vi "RaiseErrorIf.vi"(8 "error in (no error)":errorcluster, 9 "error message":string, 10 "error code (5888)":i32=5888 format="%0.0f", 11 "error? (true)":bool=TRUE) -> (0 "error out":errorcluster)   [LabVIEW 2020]
uses:
  <vilib>/Utility/error.llb/DialogType.ctl
panel:
  # "error? が true のときにエラーを生じる\n（ダイアログは出さない）\n任意のメッセージを指定できる\n（発生元情報が追加される）\nコードはデフォルトで 5888 になる"
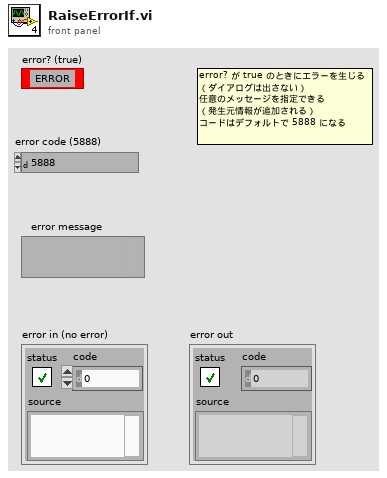
[diagram p1: front panel]
types:
  T1 = typedef "DialogType.ctl" = u16
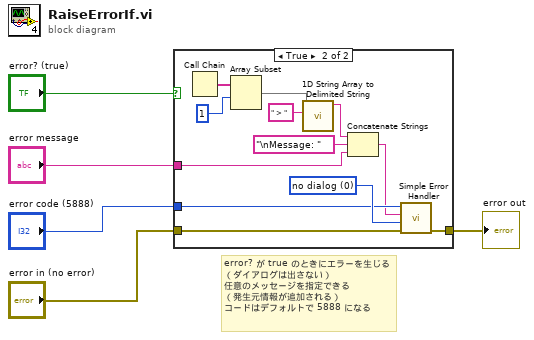
[diagram p0: block diagram]
diagram:
  # "error? が true のときにエラーを生じる\n（ダイアログは出さない）\n任意のメッセージを指定できる\n（発生元情報が追加される）\nコードはデフォルトで 5888 になる"
  n1 = case shown="True" "error? (true)" {
    tunnel: "error in (no error)" -> [w6 w18]
    tunnel: [w6 w17] -> w4
    tunnel: "error message" -> [_ w11]
    tunnel: "error code (5888)" -> [_ w15]
    frame False {
    }
    frame True {
      w16 = T1 0 items=["no dialog", "OK message", "continue or stop message", "OK message + warnings", "continue/stop + warnings"] ("type of dialog (OK msg:1)")
      n2 = Call Chain() -> (call chain=w9:string[])
      n3 = Array Subset(array=w9, index=1) -> (w7:string[])  [unwired: 1 in]
      n4 = call <vilib>:"1D String Array to Delimited String.vi"("delimiter"=" > ", "string array"=w7) -> ("delimited string"=w13:string)  [unwired: 9 in]
      n5 = Concatenate Strings(w13, "\nMessage: " ("string"), w11) -> (w10:string)
      n6 = call <vilib>:"Simple Error Handler.vi"("error code (no error:0)"=w15, "error source (\" \")"=w10, "type of dialog (OK msg:1)"=w16, "error in (no error)"=w18) -> ("error out"=w17:errorcluster)  [unwired: 1 in, 4 out]
    }
  }
  "error out" <- w4
